vi "Simulate and filter data.vi"() -> ()   [LabVIEW 2014]
panel:
  in  "Filter type":T1(ring)
  in  "Sampling Rate (Hz)":dbl=32000.0
  in  "Tab Control":enum32{"Page 1", "Page 2"}(tab)
  out "XY Graph":cluster{dbl[], "Filtered QPD data":dbl[]}[](graph)
  out "Waveform Graph 2":dbl[](graph)
  out "size(s)":i32
  out "Sampling rate after filtering (Hz)":dbl
  in  "Avg points":i32=100
  in  "#Data":i32=32000
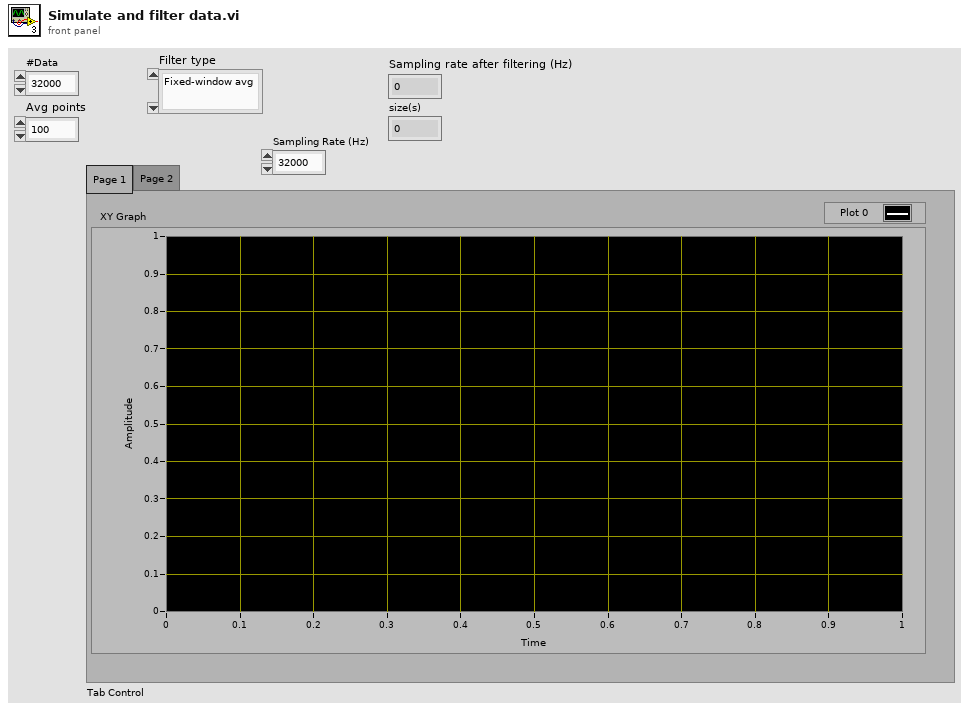
[diagram p1: front panel]
types:
  T1 = enum16{"Fixed-window avg", "Moving-window avg", "F+S-window avg", "S-G filter", "Fixed-window Median", "Moving-window Median "}
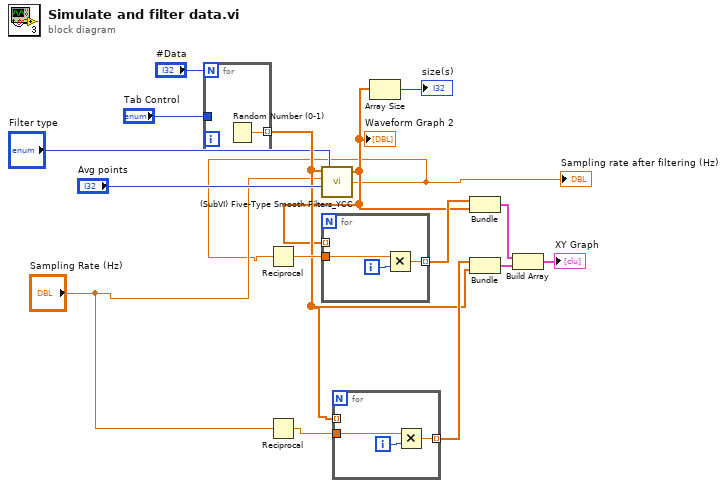
[diagram p0: block diagram]
diagram:
  n1 = for {
    N: "#Data" -> [_]
    tunnel: [w17] -> w5 mode=indexing
    tunnel: "Tab Control" -> [_]
    n2 = Random Number (0-1)() -> (number: 0 to 1=w17:dbl)
  }
  n3 = Reciprocal(x="Sampling Rate (Hz)") -> (1/x=w7:dbl)
  n4 = call "(SubVI) Five-Type Smooth Filters_YCC.vi"("Filter type"="Filter type", "Avg points"="Avg points", "Sampling rate (Hz)"="Sampling Rate (Hz)", "QPD data"=w5) -> ("Sampling rate after filtering (Hz)"=w1:dbl, "Filtered QPD data"=w4:dbl[])  [unwired: 1 in]
  "Sampling rate after filtering (Hz)" <- w1
  "Waveform Graph 2" <- w4
  n5 = Reciprocal(x=w1) -> (1/x=w13:dbl)
  n6 = for {
    tunnel: w13 -> [w20]
    tunnel: [w18] -> w12 mode=indexing
    tunnel: w4 -> [_] mode=indexing
    i -> [w19]
    n7 = Multiply(x=w20, y=w19) -> (x*y=w18:dbl)
  }
  n8 = for {
    tunnel: w7 -> [w23]
    tunnel: [w21] -> w6 mode=indexing
    tunnel: w5 -> [_] mode=indexing
    i -> [w22]
    n9 = Multiply(x=w23, y=w22) -> (x*y=w21:dbl)
  }
  n10 = Array Size(array=w4) -> (size(s)=→"size(s)":i32)
  n11 = Bundle(w12, "Filtered QPD data"=w4) -> (w8:cluster{dbl[], "Filtered QPD data":dbl[]})  [unwired: 1 in]
  n12 = Bundle(w6, w5) -> (w9:cluster{dbl[], dbl[]})  [unwired: 1 in]
  n13 = Build Array(w8, w9) -> (→"XY Graph":cluster{dbl[], "Filtered QPD data":dbl[]}[])
